vi "preparebinaryfiles.vi"(2 "filename prefix":string, 3 "data dir":path=path "C:/Users/Labmember/Desktop/Data/temp" caption="data dir.", 4 "timestamp":timestamp) -> (1 "full-filename":string)   [LabVIEW 2015]
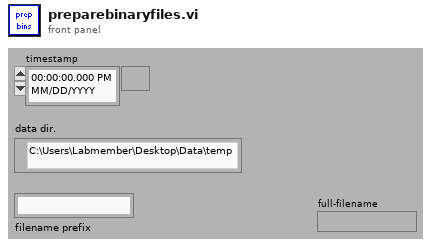
[diagram p1: front panel]
types:
  T1 = enum16{"big-endian, network order", "native, host order", "little-endian"}
  T2 = enum16{"open", "replace", "create", "open or create", "replace or create", "replace or create with confirmation"}
  T3 = typedef "LVRectTypeDef.ctl" = cluster{"Left":i16, "Top":i16, "Right":i16, "Bottom":i16}
  T4 = cluster{"Xpixels":i32, "Vxminref":dbl, "Vxmaxref":dbl, "P":dbl, "Ypixels":i32, "Vyminref":dbl, "Vymaxref":dbl, "srate":sgl, "sAOxy":i32, "timeout":dbl, "type":string, "date":string, "time":string, "Colormap":u16, "Drawing Mode":u16, "Scanning Mode":u16, "square pixels":bool, "square matrix":bool, "Xpixels Img":i32, "Vx-min Img":dbl, "VX-max Img":dbl, "Ypixels Img":i32, "Vy-min Img":dbl, "Vy-max Img ":dbl, "Angle Img":dbl, "autoshutter":bool, "finite":bool, "cont":bool, "wavdet":bool, "measpoints":i32, "avpp":i32, "bufferAO":i32, "bufferAI":i32, "starttick":u32, "waveform":path, "Vx-ref":dbl, "Vy-ref":dbl, "refreshrate":dbl, "refreshbuffer":i32, "tt_cycles":i32, "motorref":refnum<k7>, "mirrorswitch":refnum<k7>, "sample mode":i32, "maxbufferAI":i32, "srateAODO":sgl, "bin":sgl, "Pel":sgl, "Angle draw":dbl, "srate Img":sgl, "ROIimg_plotbounds":T3, "auto OD":bool, "ODfilt":u16, "aAI":i32[], "aCI":i32[], "aAO":u32[], "aDO":u32[], "refwfsize":dbl, "Lifetime":bool, "Vz-Img":dbl, "Vz-ref":dbl, "Vz-reset":dbl, "AIoverride":bool}
  T5 = cluster{"StageS":i32, "StageL":i32, "currmeas data dir":path, "image OD":u16, "contour OD":u16, "point OD":u16, "AOlines":tag[], "AIlines":tag[], "CI lines":tag[], "DO lines":tag[], "AO names":string[], "CI names":string[], "AI names":string[], "DO names":string[], "CIextensions":string[], "AIextensions":string[], "Voltage to Ygalvo":i32, "Voltage to Xgalvo":i32, "Voltage to patch":i32, "640 shutter":i32, "2P shutter":i32, "LT timestamp":u32, "Vp":i32, "Ip":i32, "camera trigger":i32, "master data dir":path, "voltage to Zpos":i32, "Vto2P":i32, "640 AO":i32, "488 AO":i32, "532 AO":i32, "640TTL":u32, "488TTL":u32, "532TTL":u32, "Device 1 sampleclock out":tag, "Device 1 Starttrigger out":tag, "Device 2 sampleclock in":tag, "Device 2 StartTrigger in ":tag, "2PODTTL":u32, "488 shutter":u32, "LCVR red":u32, "LCVR blue":u32}
  T6 = cluster{" AI":refnum<k21>, "E_AI":errorcluster, "header":dbl[]}
  T7 = cluster{"E_binfile":errorcluster[], "binfile":refnum<file>[]}
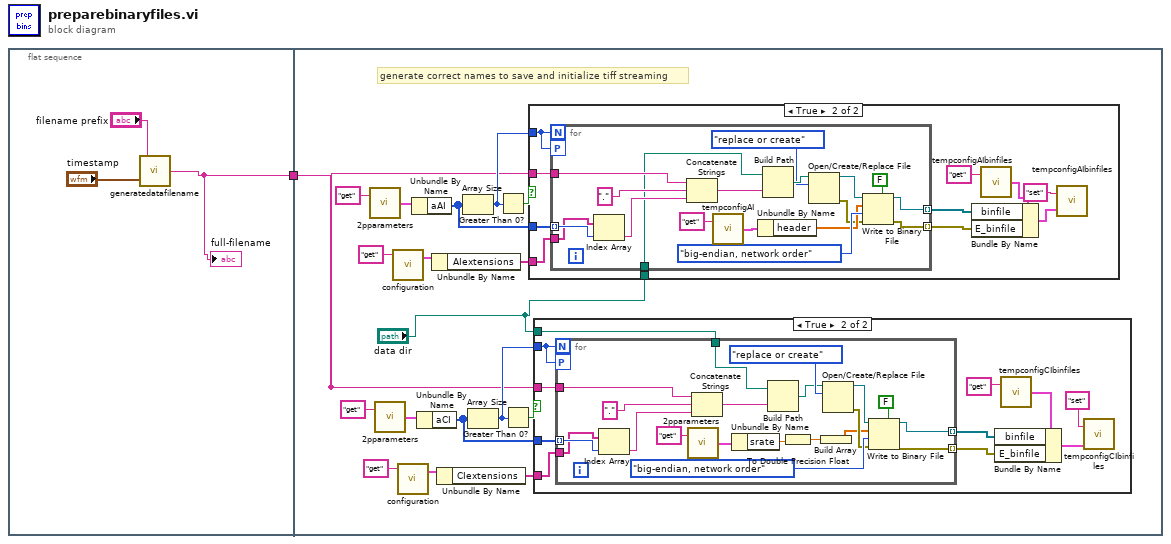
[diagram p0: block diagram]
diagram:
  n1 = flat-sequence {
    tunnel: [w2] -> w1
    tunnel: w1 -> [w6]
    frame #0 {
      n2 = call "generatedatafilename.vi"("timestamp"="timestamp", "filename prefix in"="filename prefix") -> ("full-filename"=w2:string)
      "full-filename" <- w2
    }
    frame #1 {
      # "generate correct names to save and initialize tiff streaming"
      n3 = call "2pparameters.vi"("command"="get") -> ("params out"=w22:T4)  [unwired: 1 in]
      n4 = call "2pparameters.vi"("command"="get") -> ("params out"=w7:T4)  [unwired: 1 in]
      n5 = call "configuration.vi"("command"="get") -> ("config out"=w20:T5)  [unwired: 2 in, 1 out]
      n6 = call "configuration.vi"("command"="get") -> ("config out"=w9:T5)  [unwired: 2 in, 1 out]
      n7 = Unbundle By Name(w22) -> ("aAI"=w16:i32[])
      n8 = Unbundle By Name(w7) -> ("aCI"=w13:i32[])
      n9 = Unbundle By Name(w20) -> ("AIextensions"=w15:string[])
      n10 = Unbundle By Name(w9) -> ("CIextensions"=w14:string[])
      n11 = Array Size(array=w16) -> (size(s)=w17:i32)
      n12 = Array Size(array=w13) -> (size(s)=w12:i32)
      n13 = Greater Than 0?(x=w17) -> (x > 0?=w18:bool)
      n14 = Greater Than 0?(x=w12) -> (x > 0?=w11:bool)
      n15 = case shown="True" w18 {
        tunnel: w17 -> [_ w64]
        tunnel: w16 -> [_ w63]
        tunnel: w15 -> [_ w62]
        tunnel: w6 -> [_ w59]
        tunnel: "data dir" -> [_ w58]
        frame False {
        }
        frame True {
          n16 = for {
            N: w64 -> [_]
            workers-P: w64 -> [_]
            tunnel: w63 -> [w80] mode=indexing
            tunnel: w62 -> [w79]
            tunnel: w59 -> [w77]
            tunnel: w58 -> [w76]
            tunnel: [w66] -> w56 mode=indexing
            tunnel: [w65] -> w55 mode=indexing
            n17 = Index Array(array=w79, index=w80) -> (element=w78:string)
            n18 = Concatenate Strings(w77, "." ("string"), w78) -> (w81:string)
            n19 = call "tempconfigAI.vi"("command"="get") -> ("Temp Config out"=w73:T6)  [unwired: 1 in]
            n20 = Unbundle By Name(w73) -> ("header"=w68:dbl[])
            n21 = Build Path(base path=w76, name or relative path=w81) -> (appended path=w75:path)
            n22 = Open/Create/Replace File(file path (use dialog)=w75, operation (0:open)=T2."replace or create") -> (refnum out=w69:refnum<file>, error out=w67:errorcluster)  [unwired: 4 in, 1 out]
            n23 = Write to Binary File(file (use dialog)=w69, data=w68, error in=w67, 5:FALSE ("prepend array or string size? (T)"), 9:T1."big-endian, network order" ("byte order (0:big-endian, network order)")) -> (refnum out=w66:refnum<file>, error out=w65:errorcluster)  [unwired: 1 in, 1 out]
          }
          n24 = call "tempconfigAIbinfiles.vi"("command"="get") -> ("Temp Config out"=w57:T7)  [unwired: 1 in]
          n25 = Bundle By Name(cluster=w57, "binfile"=w56, "E_binfile"=w55) -> (w54:T7)
          n26 = call "tempconfigAIbinfiles.vi"("Temp Config in"=w54, "command"="set") -> ()  [unwired: 1 out]
        }
      }
      n27 = case shown="True" w11 {
        tunnel: w12 -> [_ w33]
        tunnel: w13 -> [_ w32]
        tunnel: w14 -> [_ w31]
        tunnel: w6 -> [_ w30]
        tunnel: "data dir" -> [_ w28]
        frame False {
        }
        frame True {
          n28 = for {
            N: w33 -> [_]
            workers-P: w33 -> [_]
            tunnel: w32 -> [w51] mode=indexing
            tunnel: w31 -> [w50]
            tunnel: w30 -> [w48]
            tunnel: w28 -> [w47]
            tunnel: [w35] -> w25 mode=indexing
            tunnel: [w34] -> w24 mode=indexing
            n29 = Index Array(array=w50, index=w51) -> (element=w49:string)
            n30 = call "2pparameters.vi"("command"="get") -> ("params out"=w42:T4)  [unwired: 1 in]
            n31 = Concatenate Strings(w48, "." ("string"), w49) -> (w52:string)
            n32 = Unbundle By Name(w42) -> ("srate"=w41:sgl)
            n33 = Build Path(base path=w47, name or relative path=w52) -> (appended path=w45:path)
            n34 = To Double Precision Float(number=w41) -> (double precision float=w44:dbl)
            n35 = Build Array(w44) -> (w36:dbl[])
            n36 = Open/Create/Replace File(file path (use dialog)=w45, operation (0:open)=T2."replace or create") -> (refnum out=w38:refnum<file>, error out=w37:errorcluster)  [unwired: 4 in, 1 out]
            n37 = Write to Binary File(file (use dialog)=w38, data=w36, error in=w37, 5:FALSE ("prepend array or string size? (T)"), 9:T1."big-endian, network order" ("byte order (0:big-endian, network order)")) -> (refnum out=w35:refnum<file>, error out=w34:errorcluster)  [unwired: 1 in, 1 out]
          }
          n38 = call "tempconfigCIbinfiles.vi"("command"="get") -> ("Temp Config out"=w26:T7)  [unwired: 1 in]
          n39 = Bundle By Name(cluster=w26, "binfile"=w25, "E_binfile"=w24) -> (w23:T7)
          n40 = call "tempconfigCIbinfiles.vi"("Temp Config in"=w23, "command"="set") -> ()  [unwired: 1 out]
        }
      }
    }
  }
